vi "PipBoy_ReadFunctionsFromIconsFile.vi"(8 "error in (no error)":errorcluster, 10 "FileConf":T1) -> (0 "error out":errorcluster, 2 "Functions":string[](array[string]))   [LabVIEW 2014]
uses:
  ctls/PipBoy_FileConf.ctl
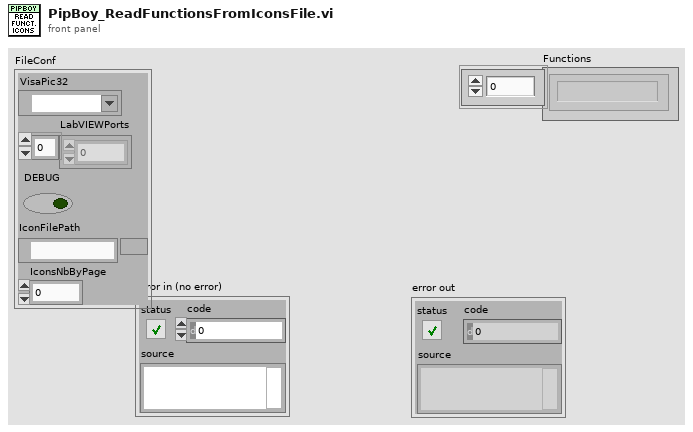
[diagram p1: front panel]
types:
  T1 = typedef "PipBoy_FileConf.ctl" = cluster{"VisaPic32":refnum<visa-resource-name>, "LabVIEWPorts":u16[], "DEBUG":bool, "IconFilePath":path, "IconsNbByPage":i32}
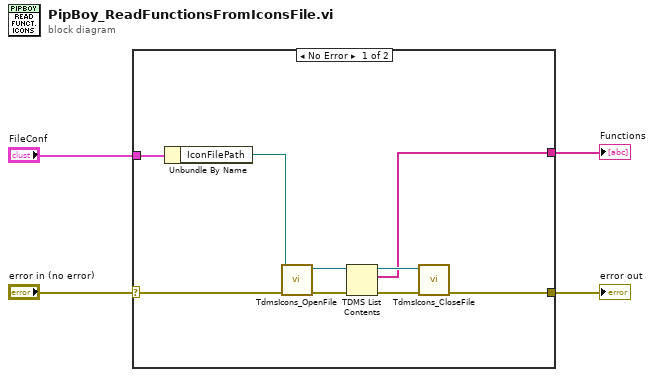
[diagram p0: block diagram]
diagram:
  n1 = case shown="No Error" "error in (no error)" {
    selector: "error in (no error)" -> [w12 w14]
    tunnel: [w8 w14] -> w3
    tunnel: "FileConf" -> [w13 _]
    tunnel: [w5 _] -> w1
    frame No Error {
      n2 = Unbundle By Name(w13) -> ("IconFilePath"=w9:path)
      n3 = call "TdmsIcons_OpenFile.vi"("error in (no error)"=w12, "Path"=w9) -> ("error out"=w11:errorcluster, "TdmsOut"=w10:refnum<k34>)  [unwired: 8 in]
      n4 = TDMS List Contents(4:w11, 7:w10) -> (0:w6:errorcluster, 2:w5:string[], 3:w7:refnum<k34>)  [unwired: 1 in, 1 out]
      n5 = call "TdmsIcons_CloseFile.vi"("error in (no error)"=w6, "TdmsIn"=w7) -> ("error out"=w8:errorcluster)  [unwired: 8 in, 1 out]
    }
    frame Error {
    }
  }
  "error out" <- w3
  "Functions" <- w1
